vi "MM9.set i attribute.vi"(0 "i ref in":refnum<vi>, 2 "i attribute":T1={"UsedObjs"=[], "ActScanStep"=[], "AbortRequest"=FALSE, "StopRequest"=FALSE, "# cycles"=0, "Connected"=FALSE, "MMStatus"=enum."config", "# data"=0, "DIMServices"={"MM6StatusString"="", "MM6StatusID"=-1, "discArchiver"="", "discArchiverID"=-1, "eventBuilder"="", "eventBuilderID"=-1, "GUIIDString"="", "GUIIDStringID"=-1}, "dataFile"="", "PGRunning"=0, "ConfigData"={"GenConfig"={"Mode"=0, "Logs"=[]}, "Configs"=[]}, "ExtraDataSets"=[]} {"ConfigData"."Configs"."CleanDev"."CleanData"."Time" format="%.3f"; "ConfigData"."Configs"."CleanDev"."CleanData"."Minus" format="%.2f"; "ConfigData"."Configs"."CleanDev"."CleanData"."Plus" format="%.2f"; "ConfigData"."Configs"."CleanDev"."CleanData"."Center" format="%.4f"; "ConfigData"."Configs"."CleanDev"."CleanData"."Amp" format="%.2f"; "ConfigData"."Configs"."Delays"."Delay" format="%.2f"; "ConfigData"."Configs"."Specials"."Data" format="%.2f"; "ConfigData"."Configs"."FreqDevs"."Time" format="%.3f"; "ConfigData"."Configs"."FreqDevs"."CenterFreq" format="%.4f"; "ConfigData"."Configs"."FreqDevs"."Amp" format="%.2f"; "ConfigData"."Configs"."Scans"."Values" format="%.2f"}, 5 "error in (no error)":errorcluster) -> (14 "i ref out":refnum<vi>, 19 "error out":errorcluster)   [LabVIEW 2014, in "MM9.lvlib"]
doc: "Sets the i attribute data of an object.\n\nLicense Agreement for this software:\n\nCopyright (C)\nGesellschaft für Schwerionenforschung, GSI\nPlanckstr. 1\n64291 Darmstadt\nGermany\n\nContact: D.Beck@gsi.de \n\nThis program is free software; you can redistribute it and/or modify it under the terms of the GNU General Public License as published by the Free Software Foundation; either version 2 of the license, or (at your option) any later version.\n\nThis program is distributed in the hope that it will be useful, but WITHOUT ANY WARRANTY; without even the implied warranty of MERCHANTABILITY or FITNESS FOR A PARTICULAR PURPOSE. See the GNU General License for more details (http://www.gnu.org).\n\nGesellschaft für Schwerionenforschung, GSI\nPlanckstr. 1, 64291 Darmstadt, Germany\nFor all questions and ideas contact: M.Richter@gsi.de, H.Brand@gsi.de or D.Beck@gsi.de.\nLast update: 17-JUN-2004"
uses:
  MM9.lvlib
  MM9.i attribute.ctl
  MM9.status.ctl
  CSDigitalIO/PPG_ABC/PPG_ABC.PG_Running.ctl
  LEBITDefs9/LEBITDefs.ConfigData.ctl
  LEBITDefs9/LEBITDefs.GenConfig.ctl
  LEBITDefs9/LEBITDefs.Log.ctl
  LEBITDefs9/LEBITDefs.OneConfig.ctl
  LEBITDefs9/LEBITDefs.MCA.ctl
  LEBITDefs9/LEBITDefs.Timing.ctl
  LEBITDefs9/LEBITDefs.Timetable.ctl
  LEBITDefs9/LEBITDefs.Memory.ctl
  LEBITDefs9/LEBITDefs.ScanDev.ctl
  LEBITDefs9/LEBITDefs.FreqDev.ctl
  LEBITDefs9/LEBITDefs.CleanDev.ctl
  LEBITDefs9/LEBITDefs.CleanDataType.ctl
  LEBITDefs9/LEBITDefs.Special.ctl
  LEBITDefs9/LEBITDefs.Delay.ctl
  LEBITDefs9/LEBITDefs.DAC.ctl
  LEBITDefs9/LEBITDefs.ExtraData.ctl
  CSDigitalIO/PPG_ABC/PPG_ABC.lvlib
  LEBITDefs9/LEBITDefs9.lvlib
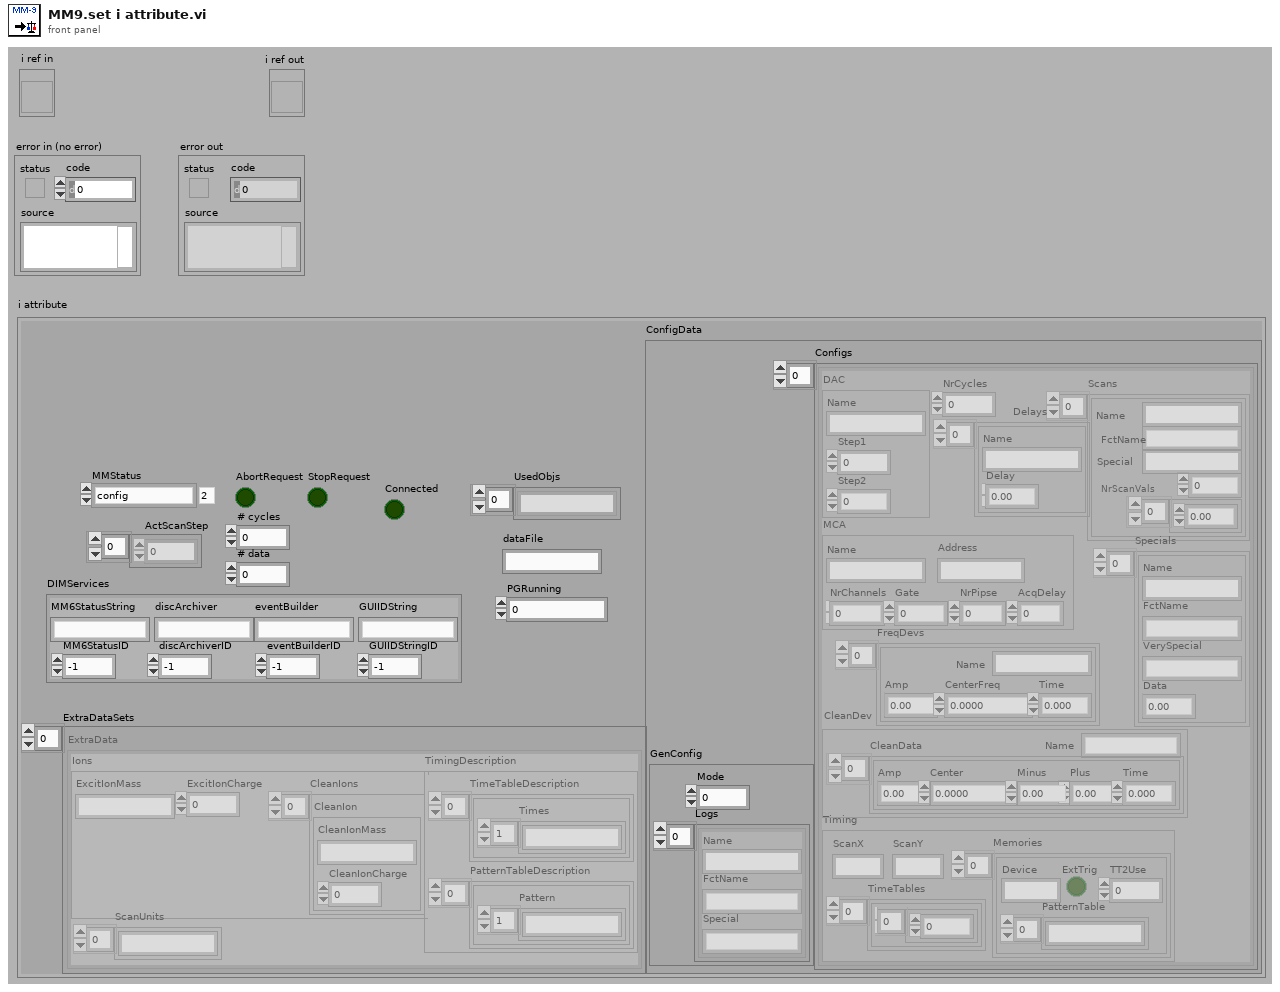
[diagram p1: front panel]
types:
  T1 = typedef "MM9.lvlib/MM9.i attribute.ctl" = cluster{"UsedObjs":string[], "ActScanStep":i32[], "AbortRequest":bool, "StopRequest":bool, "# cycles":i32, "Connected":bool, "MMStatus":T2, "# data":i32, "DIMServices":cluster{"MM6StatusString":string, "MM6StatusID":i32, "discArchiver":string, "discArchiverID":i32, "eventBuilder":string, "eventBuilderID":i32, "GUIIDString":string, "GUIIDStringID":i32}, "dataFile":string, "PGRunning":T3, "ConfigData":T4, "ExtraDataSets":T19}
  T2 = typedef "MM9.lvlib/MM9.status.ctl" = enum16{"loaded", "load_error", "config", "config_error", "init", "init_error", "data_reset", "data_reset_error", "running", "start_error", "run_error", "abort_requested", "aborted", "stop_requested", "stopped", "stop_error", "Connected", "NOTConnected"}
  T3 = typedef "PPG_ABC.lvlib/PPG_ABC.PG_Running.ctl" = i32
  T4 = typedef "LEBITDefs9.lvlib/LEBITDefs.ConfigData.ctl" = cluster{"GenConfig":T5, "Configs":T7[]}
  T5 = typedef "LEBITDefs9.lvlib/LEBITDefs.GenConfig.ctl" = cluster{"Mode":i32, "Logs":T6[]}
  T6 = typedef "LEBITDefs9.lvlib/LEBITDefs.Log.ctl" = cluster{"Name":string, "FctName":string, "Special":string}
  T7 = typedef "LEBITDefs9.lvlib/LEBITDefs.OneConfig.ctl" = cluster{"MCA":T8, "Timing":T9, "Scans":T12[], "FreqDevs":T13[], "CleanDev":T14, "NrCycles":i32, "Specials":T16[], "Delays":T17[], "DAC":T18}
  T8 = typedef "LEBITDefs9.lvlib/LEBITDefs.MCA.ctl" = cluster{"Name":string, "Address":string, "NrChannels":i32, "Gate":i32, "NrPipse":i32, "AcqDelay":i32}
  T9 = typedef "LEBITDefs9.lvlib/LEBITDefs.Timing.ctl" = cluster{"TimeTables":cluster{"TimeTable":T10}[], "Memories":T11[], "ScanX":string, "ScanY":string}
  T10 = typedef "LEBITDefs9.lvlib/LEBITDefs.Timetable.ctl" = dbl[]
  T11 = typedef "LEBITDefs9.lvlib/LEBITDefs.Memory.ctl" = cluster{"Device":string, "ExtTrig":bool, "TT2Use":i32, "PatternTable":string[]}
  T12 = typedef "LEBITDefs9.lvlib/LEBITDefs.ScanDev.ctl" = cluster{"Name":string, "FctName":string, "Values":dbl[], "NrScanVals":i32, "Special":string}
  T13 = typedef "LEBITDefs9.lvlib/LEBITDefs.FreqDev.ctl" = cluster{"Name":string, "Amp":dbl, "CenterFreq":dbl, "Time":dbl}
  T14 = typedef "LEBITDefs9.lvlib/LEBITDefs.CleanDev.ctl" = cluster{"Name":string, "CleanData":T15[]}
  T15 = typedef "LEBITDefs9.lvlib/LEBITDefs.CleanDataType.ctl" = cluster{"Amp":dbl, "Center":dbl, "Plus":dbl, "Minus":dbl, "Time":dbl}
  T16 = typedef "LEBITDefs9.lvlib/LEBITDefs.Special.ctl" = cluster{"Name":string, "FctName":string, "VerySpecial":string, "Data":dbl}
  T17 = typedef "LEBITDefs9.lvlib/LEBITDefs.Delay.ctl" = cluster{"Name":string, "Delay":dbl}
  T18 = typedef "LEBITDefs9.lvlib/LEBITDefs.DAC.ctl" = cluster{"Name":string, "Step1":i32, "Step2":i32}
  T19 = typedef "LEBITDefs9.lvlib/LEBITDefs.ExtraData.ctl" = cluster{"Ions":cluster{"ExcitIonMass":string, "ExcitIonCharge":i32, "CleanIons":cluster{"CleanIonMass":string, "CleanIonCharge":i32}[]}, "TimingDescription":cluster{"TimeTableDescription":cluster{"Times":string[]}[], "PatternTableDescription":cluster{"Pattern":string[]}[]}, "ScanUnits":string[]}[]
  T20 = enum16{"SetAttribute", "GetAttribute", "CreateAttribute", "DestroyAttribute", "DestroyAllAtributes"}
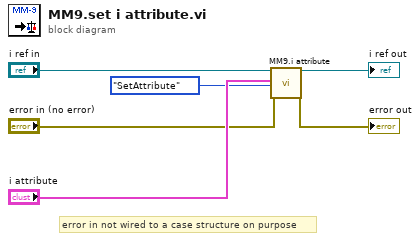
[diagram p0: block diagram]
diagram:
  # "error in not wired to a case structure on purpose"
  n1 = call "MM9.i attribute.vi"("VI Refnum"="i ref in", "CLASS.i attribute"="i attribute", "Action"=T20."SetAttribute", "error in (no error)"="error in (no error)") -> ("VI Refnum out"=→"i ref out":refnum<vi>, "error out"=→"error out":errorcluster)  [unwired: 13 in, 1 out]
